vi "2ButtonSetpointServo.vi"(8 "Setpoint B":i32=70, 9 "Setpoint A":i32=70, 10 "Button 1":bool, 11 "Button 2":bool) -> (2 "Value Out":i32=70)   [LabVIEW 2018]
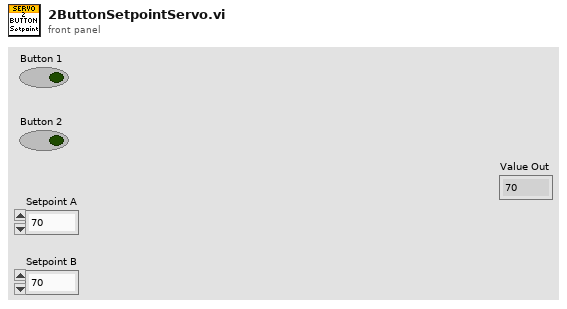
[diagram p1: front panel]
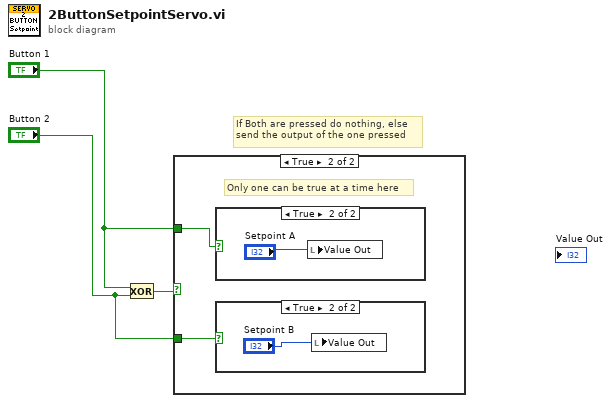
[diagram p0: block diagram]
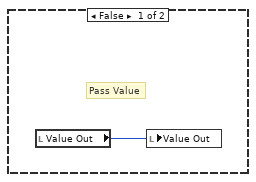
[diagram p2: hidden frame]
diagram:
  # "If Both are pressed do nothing, else\nsend the output of the one pressed"
  n1 = Exclusive Or(1:"Button 2", 2:"Button 1") -> (0:w2:bool)
  n2 = case shown="True" w2 {
    tunnel: "Button 1" -> [_ w6]
    tunnel: "Button 2" -> [_ w5]
    frame False {
      # "Pass Value"
      n3 = local read "Value Out"() -> (w4:i32)
      n4 = local write "Value Out"(w4) -> ()
    }
    frame True {
      # "Only one can be true at a time here"
      n5 = case shown="True" w6 {
        frame False {
        }
        frame True {
          n6 = local write "Value Out"("Setpoint A") -> ()
        }
      }
      n7 = case shown="True" w5 {
        frame False {
        }
        frame True {
          n8 = local write "Value Out"("Setpoint B") -> ()
        }
      }
    }
  }
